vi "D2Character - Accessors - Get Class.vi"(8 "error in (no error)":errorcluster, 11 "D2Character in":refnum<class "D2Character.lvclass">) -> (0 "error out":errorcluster, 2 "Class":T1, 3 "D2Character out":refnum<class "D2Character.lvclass">)   [LabVIEW 2015, in "D2Character.lvclass"]
uses:
  D2Character.lvclass
  D2Character - Char Class.ctl
  D2Character.lvclass/D2Character.ctl
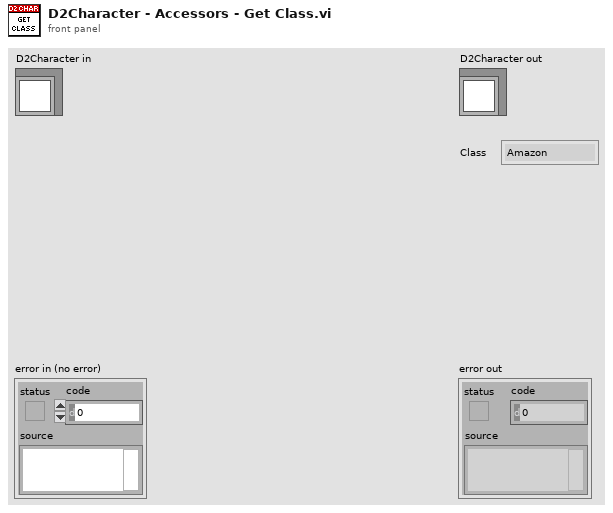
[diagram p1: front panel]
types:
  T1 = typedef "D2Character.lvclass/D2Character - Char Class.ctl" = enum8{"Amazon", "Sorceress", "Necromancer", "Paladin", "Barbarian", "Druid", "Assassin"}
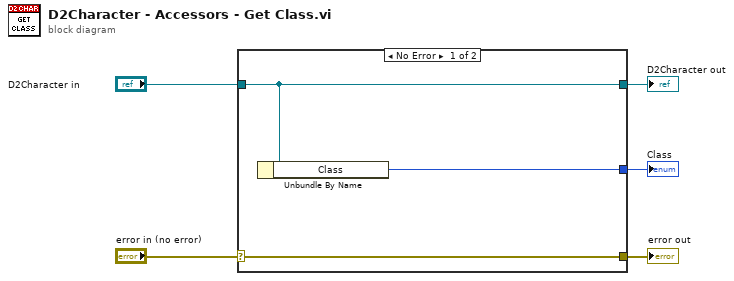
[diagram p0: block diagram]
diagram:
  n1 = case shown="No Error" "error in (no error)" {
    selector: "error in (no error)" -> [w8 w9]
    tunnel: [w8 w9] -> w4
    tunnel: [w7 w10] -> w2
    tunnel: "D2Character in" -> [w7 w10]
    tunnel: [w6 _] -> w1
    frame No Error {
      n2 = Unbundle By Name(w7) -> ("Class"=w6:T1)
    }
    frame Error {
    }
  }
  "error out" <- w4
  "D2Character out" <- w2
  "Class" <- w1
